vi "LockInArduino Final.vi"() -> ()   [LabVIEW 2018]
uses:
  <vilib>/LabVIEW Interface for Arduino/Type Defs/Analog Pin.ctl
  <vilib>/Analysis/NI_AALPro.lvlib
  <vilib>/LabVIEW Interface for Arduino/LabVIEW Interface for Arduino.lvlib
panel:
  out "Data 7":waveform(dbl)(graph)
  in  "Frequency 2":u16=500 step=100
  in  "Buzzer Switch 2":bool
  in  "Tone DO Pin 2":u8=8
  in  "Duration ms 2":u32=1
  out "Data 6":waveform(dbl)[](graph)
  in  "Number of Samples 3":u16
  in  "Acquition Speed (HZ) 3":u16
  in  "Analog Pin 3":T1
  out "Data 4":waveform(dbl)[](graph)
  out "Amplitude History":dbl(graph)
  out "θ":dbl
  out "R":dbl
  out "Error Out":errorcluster caption="Error"
  in  "Stop":bool
  out "Y":dbl
  out "X":dbl
  out "# of elements in queue":i32
  in  "Allowance":dbl=0.1
  # "Allowance means presicision of PLL\nPlease set this as positive value (>0)\nThe little the value is, the presicision will be good but\nit take more time to settle."
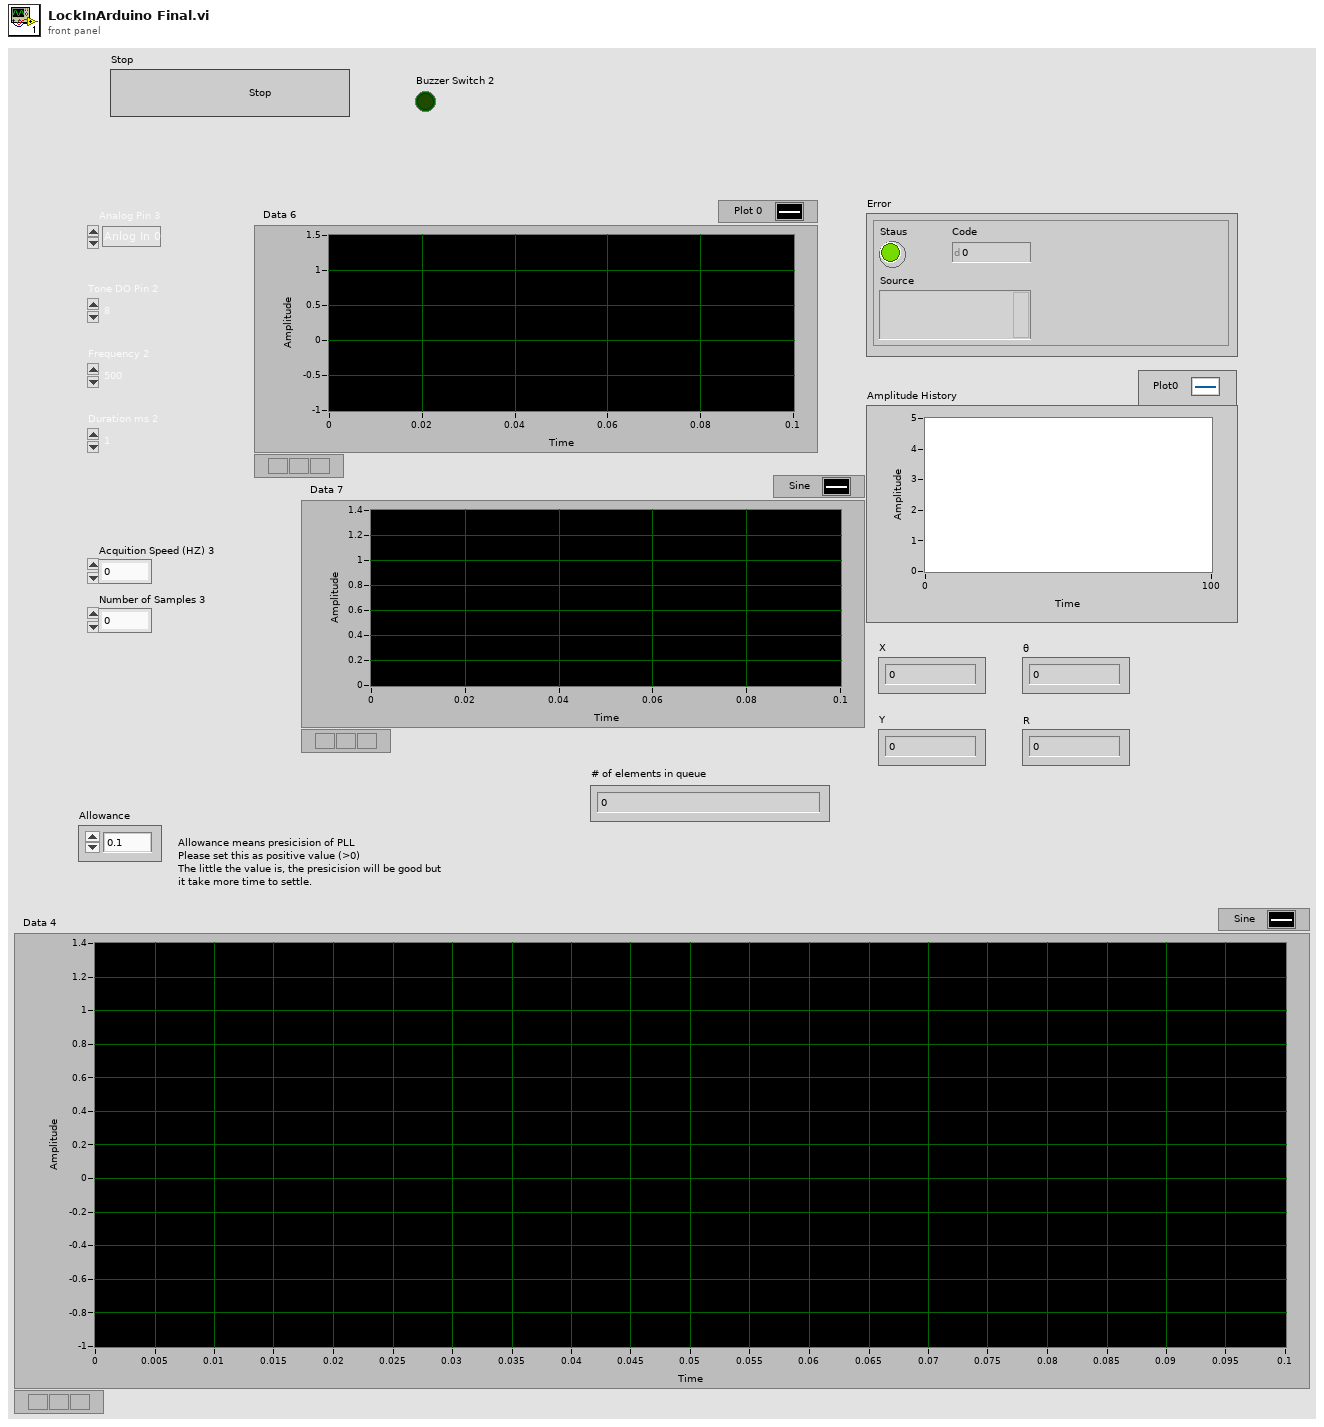
[diagram p1: front panel]
types:
  T1 = typedef "LabVIEW Interface for Arduino.lvlib/Analog Pin.ctl" = enum8{"Anlog In 0", "Anlog In 1", "Anlog In 2", "Anlog In 3", "Anlog In 4", "Anlog In 5"}
  T2 = typedef "LabVIEW Interface for Arduino.lvlib/Arduino Resource.ctl" = cluster{"VISA resource":refnum<visa-resource-name>, "Board Type":T3, "Connection Type":enum8{"USB / Serial"}, "Bytes Per Packet (15)":u8}
  T3 = typedef "LabVIEW Interface for Arduino.lvlib/Board Type.ctl" = enum16{"Uno", "Dimuelanove w/Atmega 328", "Mega 2560"}
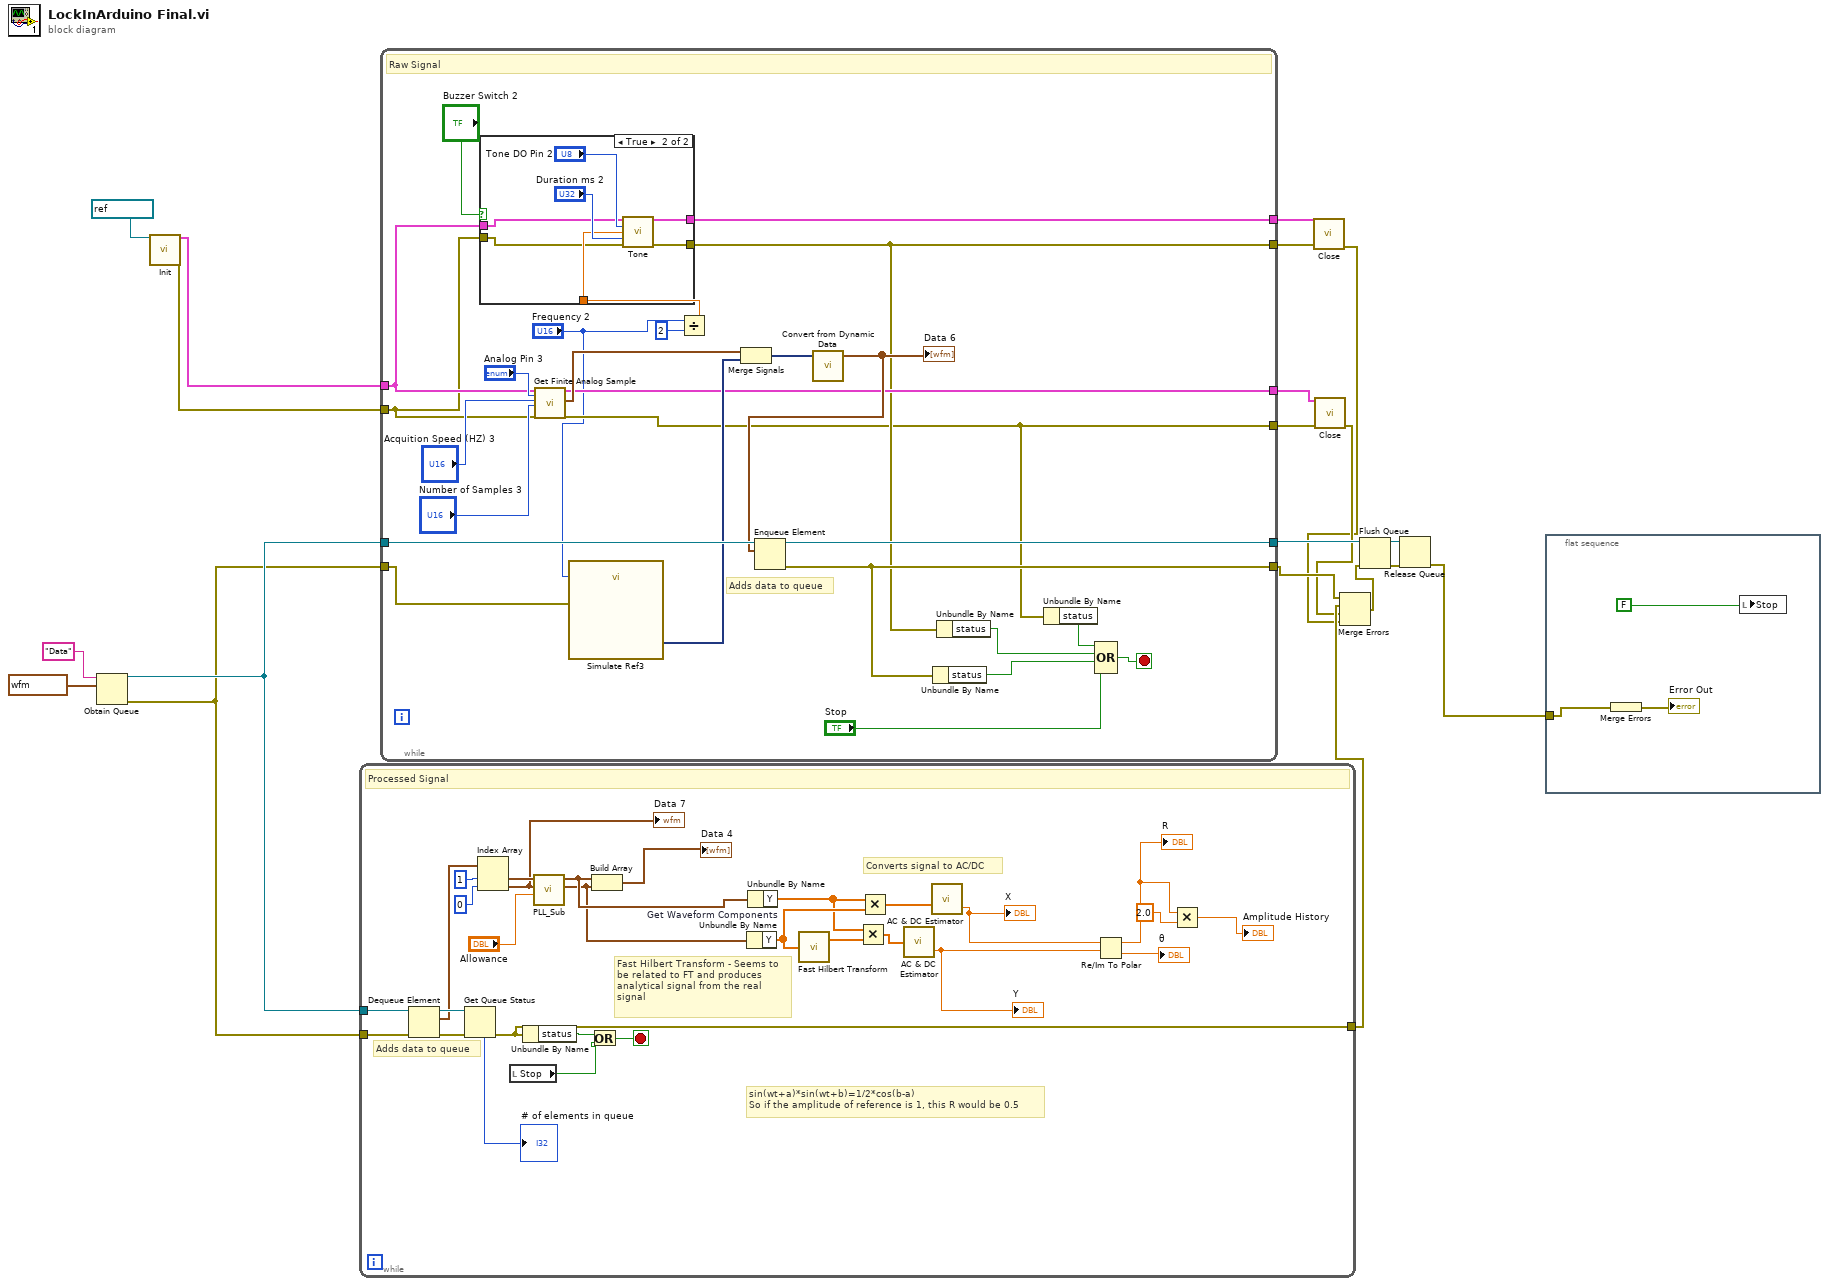
[diagram p0: block diagram]
diagram:
  n1 = Obtain Queue(name (unnamed)="Data" ("名前（名前なし）"), element data type=waveform(dbl)[] [{"t0"=timestamp(3571029634.6453953 s since 1904-01-01), "dt"=1.9999999999999998e-05, "Y"=array[5000 elements]}, {"t0"=timestamp(3571029634.6453953 s since 1904-01-01), "dt"=1.9999999999999998e-05, "Y"=array[5000 elements]}] ("計測波形")) -> (queue out=w18:refnum<queue>, error out=w17:errorcluster)  [unwired: 3 in, 1 out]
  n2 = call <vilib>:"Init.vi"("VISA resource"=refnum<visa-resource-name> "COM4") -> ("Arduino Resource"=w8:T2, "error out"=w7:errorcluster)  [unwired: 17 in]
  n3 = while {
    tunnel: w18 -> [w48]
    tunnel: w17 -> [w47]
    tunnel: [w39] -> w11
    stop <- w40 stop-if-true
    # "Converts signal to AC/DC"
    # "Adds data to queue"
    # "sin(wt+a)*sin(wt+b)=1/2*cos(b-a)\nSo if the amplitude of reference is 1, this R would be 0.5"
    # "Fast Hilbert Transform - Seems to be related to FT and produces analytical signal from the real signal"
    # "Processed Signal"
    n4 = Dequeue Element(queue=w48, error in (no error)=w47) -> (queue out=w46:refnum<queue>, element=w44:waveform(dbl)[], error out=w45:errorcluster)  [unwired: 1 in, 1 out]
    n5 = Get Queue Status(queue=w46, error in (no error)=w45) -> (error out=w39:errorcluster, # elements in queue=→"# of elements in queue":i32)  [unwired: 1 in, 6 out]
    n6 = Index Array "Index Array"(array=w44, index #1=1 ("指標"), index #2=0 ("指標")) -> (element #1=w22:waveform(dbl), element #2=w21:waveform(dbl))
    "Data 7" <- w21
    n7 = local read "Stop"() -> (w30:bool)
    n8 = Unbundle By Name(w39) -> ("status"=w41:bool)
    n9 = call "PLL_Sub.vi"("Allowance"="Allowance", "Sig"=w21, "Ref"=w22) -> ("Sig Out Feed through"=w31:waveform(dbl), "Ref_PLL_Out"=w32:waveform(dbl))  [unwired: 7 in]
    n10 = Or(x=w41, y=w30) -> (x .or. y?=w40:bool)
    n11 = Build Array "Build Array"(w32, w31) -> (→"Data 4":waveform(dbl)[])
    n12 = Unbundle By Name(w31) -> ("Y"=w36:dbl[])
    n13 = Unbundle By Name "Get Waveform Components"(w32) -> ("Y"=w35:dbl[])
    n14 = call <vilib>:"Fast Hilbert Transform.vi"("X"=w36) -> ("Hilbert{X}"=w37:dbl[])  [unwired: 1 out]
    n15 = Multiply(x=w35, y=w37) -> (x*y=w33:dbl[])
    n16 = Multiply(x=w35, y=w36) -> (x*y=w34:dbl[])
    n17 = call <vilib>:"AC & DC Estimator.vi"("Signal (V)"=w33) -> ("DC estimate (V)"=w28:dbl)  [unwired: 1 out]
    "Y" <- w28
    n18 = call <vilib>:"AC & DC Estimator.vi"("Signal (V)"=w34) -> ("DC estimate (V)"=w29:dbl)  [unwired: 1 out]
    "X" <- w29
    n19 = Re/Im To Polar(2:w28, 3:w29) -> (0:→"θ":dbl, 1:w26:dbl)
    "R" <- w26
    n20 = Multiply(x=w26, y=2.0) -> (x*y=→"Amplitude History":dbl)
  }
  n21 = while {
    tunnel: w18 -> [w75]
    tunnel: w17 -> [w62]
    tunnel: [w74] -> w15
    tunnel: [w73] -> w12
    tunnel: w8 -> [w60]
    tunnel: w7 -> [w59]
    tunnel: [w58] -> w5
    tunnel: [w54] -> w4
    tunnel: [w57] -> w3
    tunnel: [w56] -> w2
    stop <- w71 stop-if-true
    # "Adds data to queue"
    # "4."
    # "Raw Signal"
    n22 = call <vilib>:"Get Finite Analog Sample.vi"("Arduino Resource"=w60, "Analog Input Pin"="Analog Pin 3", "Acquition Speed (HZ)"="Acquition Speed (HZ) 3", "Number of Samples"="Number of Samples 3", "error in"=w59) -> ("Arduino Resource"=w58:T2, "Data"=w65:waveform(dbl), "error out"=w54:errorcluster)  [unwired: 11 in, 1 out]
    n23 = call "Simulate Ref3"("Frequency"="Frequency 2", "error in (no error)"=w62) -> ("Sine"=w66:dynamicdata)  [unwired: 12 in, 1 out]
    n24 = Divide(x="Frequency 2", y=u16 2) -> (x/y=w52:dbl)
    n25 = case shown="True" "Buzzer Switch 2" {
      tunnel: [w77 w84] -> w57
      tunnel: [w76 w83] -> w56
      tunnel: w52 -> [_ w80]
      tunnel: w60 -> [w77 w79]
      tunnel: w59 -> [w76 w78]
      frame False {
      }
      frame True {
        n26 = call <vilib>:"Tone.vi"("Arduino Resource"=w79, "Tone DO Pin"="Tone DO Pin 2", "Frequency (0 Hz)"=w80, "Duration (1 ms)"="Duration ms 2", "error in"=w78) -> ("Arduino Resource"=w84:T2, "error out"=w83:errorcluster)  [unwired: 9 in]
      }
    }
    n27 = Merge Signals(w65, w66) -> (w64:dynamicdata)
    n28 = call "Convert from Dynamic Data"("Dynamic Data Type"=w64) -> ("Array of Waveform"=w61:waveform(dbl)[])  [unwired: 3 in]
    "Data 6" <- w61
    n29 = Enqueue Element(queue=w75, element=w61) -> (queue out=w74:refnum<queue>, error out=w73:errorcluster)  [unwired: 2 in, 1 out]
    n30 = Unbundle By Name "Unbundle By Name"(w73) -> ("status"=w72:bool)
    n31 = Unbundle By Name "Unbundle By Name"(w56) -> ("status"=w55:bool)
    n32 = Unbundle By Name "Unbundle By Name"(w54) -> ("status"=w53:bool)
    n33 = Compound Arithmetic op=OR ("複合演算")(w53, w55, w72, "Stop") -> (w71:bool)
  }
  n34 = call <vilib>:"Close.vi"("Arduino Resource"=w3, "error in"=w2) -> ("error out"=w1:errorcluster)  [unwired: 13 in]
  n35 = call <vilib>:"Close.vi"("Arduino Resource"=w5, "error in"=w4) -> ("error out"=w6:errorcluster)  [unwired: 13 in]
  n36 = Merge Errors(w12, w11, w6, w1) -> (w10:errorcluster)
  n37 = Flush Queue(queue=w15, error in (no error)=w10) -> (queue out=w13:refnum<queue>, error out=w14:errorcluster)  [unwired: 1 out]
  n38 = Release Queue(queue=w13, error in (no error)=w14) -> (error out=w16:errorcluster)  [unwired: 1 in, 2 out]
  n39 = flat-sequence {
    tunnel: w16 -> [w85]
    frame #0 {
      n40 = Merge Errors(w85) -> (→"Error Out":errorcluster)
      n41 = local write "Stop"(FALSE ("停止")) -> ()
    }
  }
